vi "Binary-record-&-read.vi"   [LabVIEW 2015]
uses:
  <vilib>/Platform/TimedLoop/XDataNode/timing_clust.ctl
  <vilib>/Platform/TimedLoop/XDataNode/nitl_modes.ctl
  <vilib>/Platform/TimedLoop/XDataNode/wakeup.ctl
  <vilib>/Rock Robotics/WPI/Utilities/WPI_GetSetVariantRefNum.vi
  Robot Global Data.vi
  <vilib>/platform/TimedLoop/XDataNode/XDataNode.xnode
  <vilib>/Platform/TimedLoop/XDataNode/XDNodeRunTimeDep.lvlib
types:
  T1 = typedef "WPI_MotorControlDeviceRef.ctl" = cluster{"DeviceStatus":errorcluster, "Type":T2, "PWM":cluster{"PWM Channel":T3, "DeadBand":T4}, "CAN":cluster{"Device Number":u8, "Control Mode":T5, "Semaphore":T6, "Max Vout":dbl, "TalonSRX Control Mode":T7}, "Invert":bool}
  T2 = typedef "WPI_MotorControlType.ctl" = enum16{"PWM", "CAN", "CANTalonSRX"}
  T3 = typedef "FPGA_DIOPWMChannel.ctl" = enum8{"PWM 0", "PWM 1", "PWM 2", "PWM 3", "PWM 4", "PWM 5", "PWM 6", "PWM 7", "PWM 8", "PWM 9", "PWM MXP 0", "PWM MXP 1", "PWM MXP 2", "PWM MXP 3", "PWM MXP 4", "PWM MXP 5", "PWM MXP 6", "PWM MXP 7", "PWM MXP 8", "PWM MXP 9", "Invalid"}
  T4 = typedef "WPI_PWMDeadband.ctl" = cluster{"Name":string, "maxPositivePwm":i32, "minPositivePwm":i32, "centerPwm":i32, "maxNegativePwm":i32, "minNegativePwm":i32, "angularRange":u16}
  T5 = typedef "WPI_CANJaguar_ControlMode.ctl" = enum8{"Percent VBus", "Current", "Speed", "Position", "Voltage"}
  T6 = typedef "Semaphore RefNum" = refnum<k1>
  T7 = typedef "WPI_CANTalonSRX_APIControlMode.ctl" = enum8{"Percent VBus", "Speed", "Position", "Slave", "Unchanged / Invalid", "Voltage Compensation", "Current", "Motion Profile"}
  T8 = typedef "WPI_JoystickDevRef.ctl" = cluster{"Device":T9}
  T9 = typedef "WPI_JoystickDeviceEnum.ctl" = enum16{"USB 0", "USB 1", "USB 2", "USB 3", "USB 4", "USB 5"}
  T10 = typedef "XDNodeRunTimeDep.lvlib/timing_clust.ctl" = cluster{"Expected End [f-1]":u64, "Actual End [f-1]":u64, "Finished Late? [f-1]":bool, "Expected End [i-1]":u64, "Actual End [i-1]":u64, "Finished Late? [i-1]":bool, "Expected Start [i]":u64, "Actual Start [i]":u64, "Expected Start [f]":u64, "Actual Start [f]":u64, "Source Name":string, "Structure Name":string, "Period":i64, "Deadline":i64, "Offset":i64, "Start":i64, "Priority":i32, "Timeout":i32, "Mode":T11, "Wakeup Reason":T12, "Error":errorcluster, "Source Type":string, "Secondary Source Type":string, "Global End Time":u64, "Global Start Time":u64, "Frame Duration":u64, "Iteration Duration":u64, "Assigned CPU":i32, "I/O Scan Engine Mode":u32}
  T11 = typedef "XDNodeRunTimeDep.lvlib/nitl_modes.ctl" = enum32{"No Change", "Process missed periods, maintain original phase", "Discard missed periods, maintain original phase", "Process missed periods, ignore original phase", "Discard missed periods, ignore original phase"}
  T12 = typedef "XDNodeRunTimeDep.lvlib/wakeup.ctl" = enum32{"Normal", "Aborted", "Asynchronous wakeup", "Timing source error", "Timed loop error", "Timeout"}
  T13 = enum16{"open", "replace", "create", "open or create", "replace or create", "replace or create with confirmation"}
  T14 = enum16{"open", "open or create", "create or replace", "create", "open (read-only)"}
  T15 = cluster{"Record?":bool, "Current File":string, "Run script?":bool, "Stop recording?":bool, "Stop script?":bool}
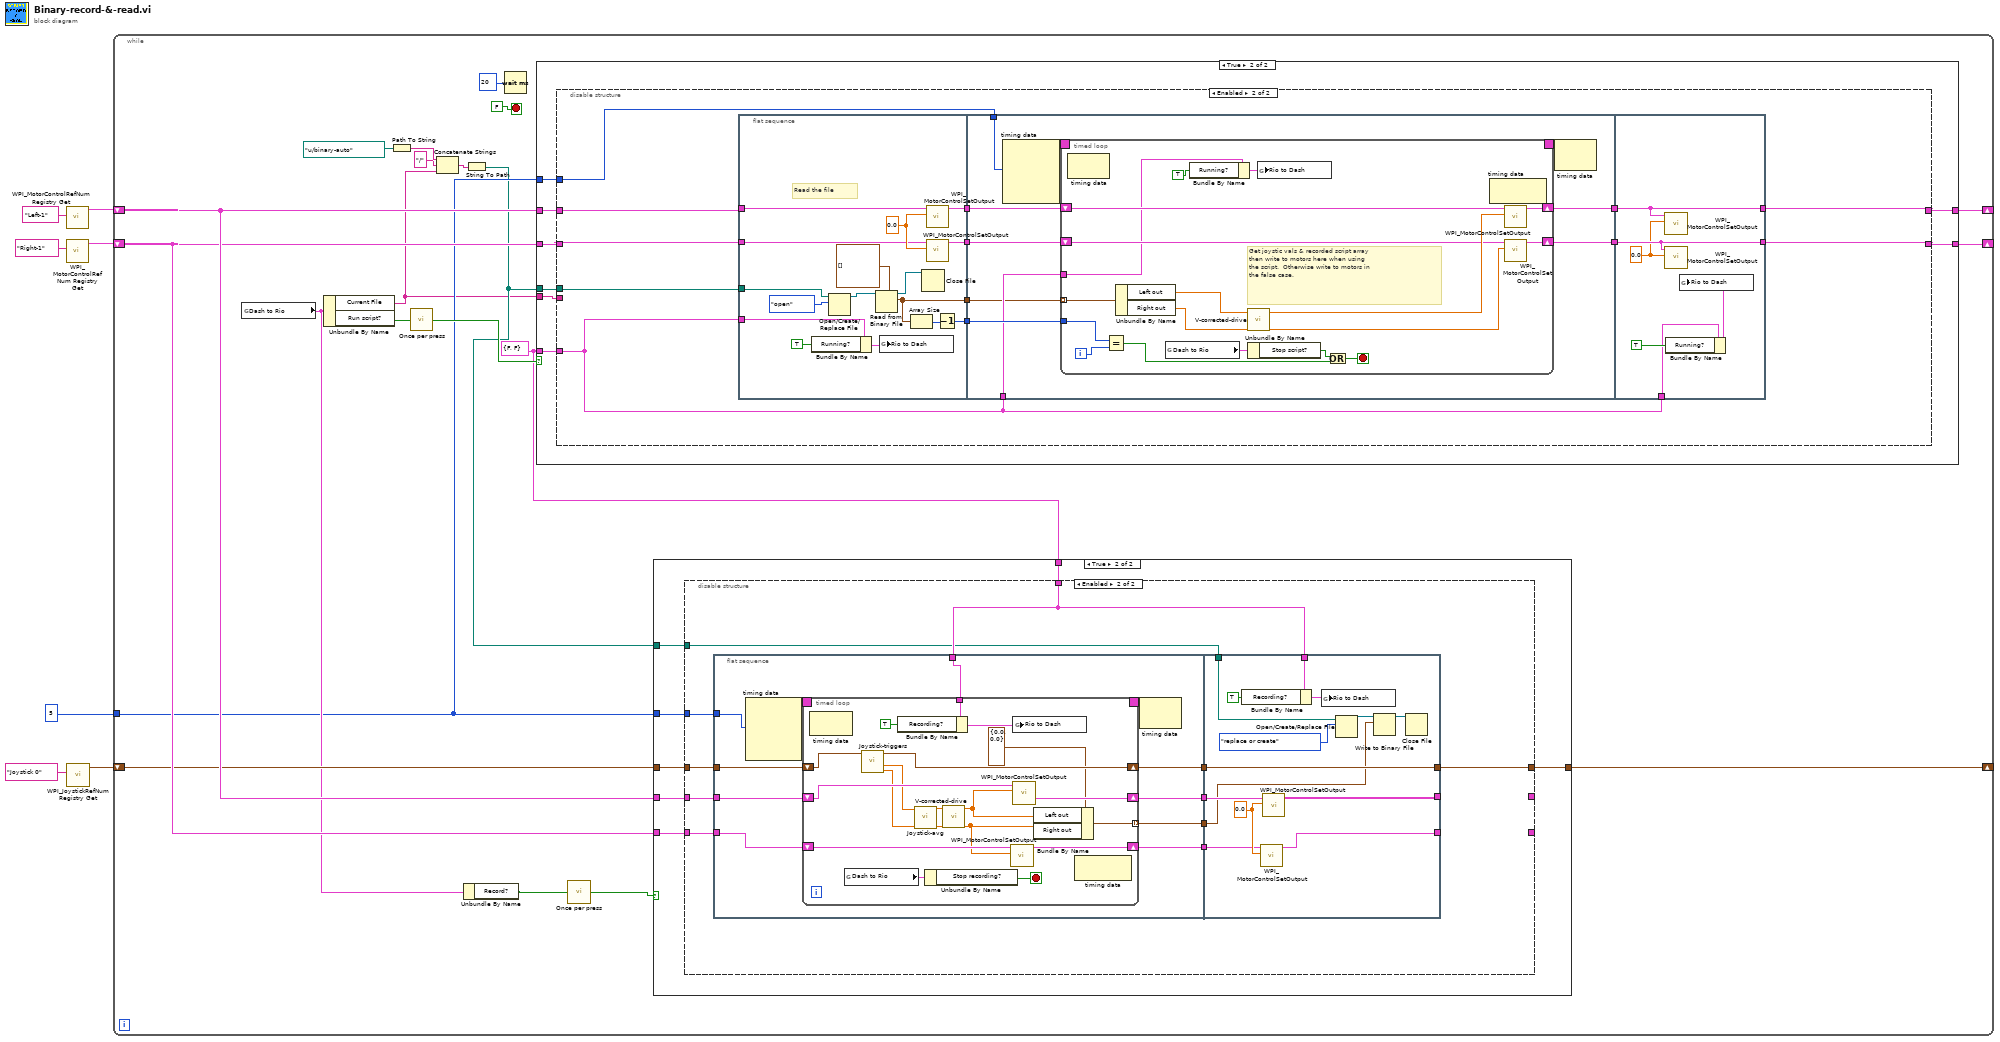
[diagram p0: block diagram]
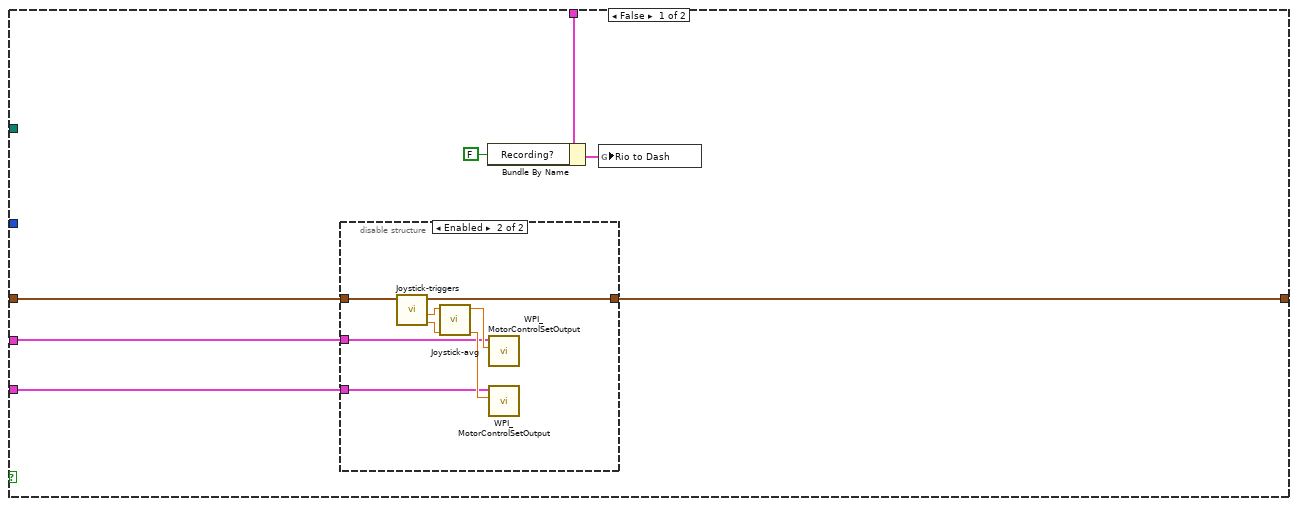
[diagram p2: hidden frame]
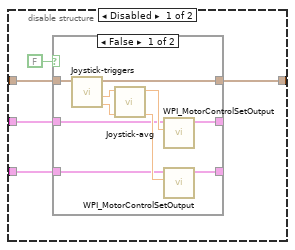
[diagram p3: hidden frame]
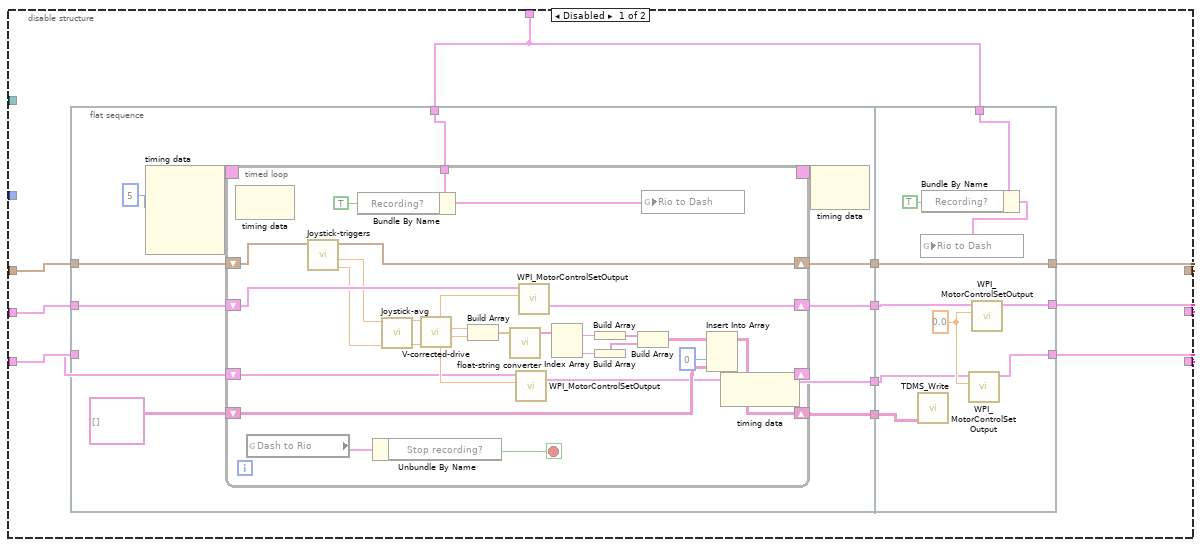
[diagram p5: hidden frame]
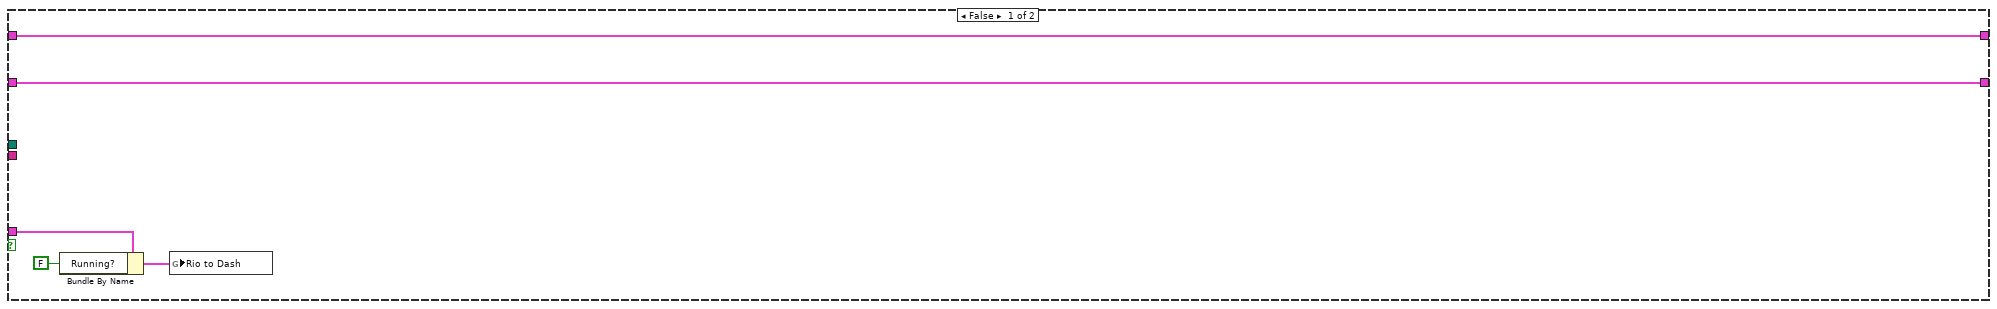
[diagram p6: hidden frame]
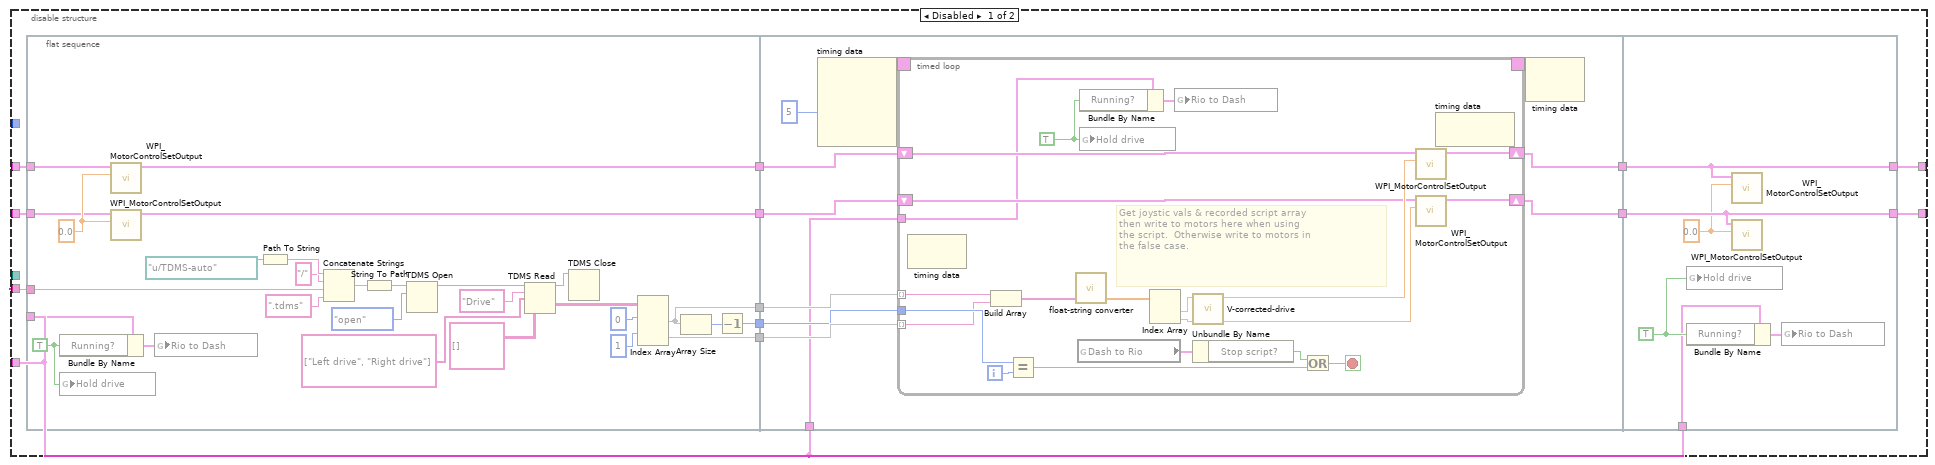
[diagram p7: hidden frame]
diagram:
  n1 = call <vilib>:"WPI_MotorControlRefNum Registry Get.vi"("refnum name"="Left-1") -> ("MotorControlDevRef"=w4:T1)  [unwired: 9 in, 1 out]
  n2 = call <vilib>:"WPI_MotorControlRefNum Registry Get.vi"("refnum name"="Right-1") -> ("MotorControlDevRef"=w5:T1)  [unwired: 9 in, 1 out]
  n3 = call <vilib>:"WPI_JoystickRefNum Registry Get.vi"("refnum name"="Joystick 0") -> ("JoystickDevRef"=w2:T8)  [unwired: 1 in, 9 out]
  n4 = while {
    shift-right: [w26] -> _
    shift-left: w5 -> [w20]
    shift-right: [w25] -> _
    shift-left: w4 -> [w21]
    shift-right: [w19] -> _
    shift-left: w2 -> [w18]
    tunnel: i64 5 ("Period") -> [w15]
    stop <- FALSE stop-if-true
    w16 = cluster{"Recording?":bool, "Running?":bool} {"Recording?"=FALSE, "Running?"=FALSE} ("Rio to Dash")
    n5 = global read "Robot Global Data.vi" "Dash to Rio"() -> (w17:T15)
    n6 = Unbundle By Name(w17) -> ("Current File"=w9:string, "Run script?"=w23:bool)
    n7 = Path To String(path=path "u:/binary-auto" ("file path 3")) -> (string=w13:string)
    n8 = call "Once per press.vi"("In"=w23) -> ("Out"=w24:bool)  [unwired: 2 in]
    n9 = Concatenate Strings(w13, "/" ("string"), w9) -> (w12:string)
    n10 = Unbundle By Name(w17) -> ("Record?"=w22:bool)
    n11 = String To Path(string=w12) -> (path=w10:path)
    n12 = Wait (ms)(milliseconds to wait=u32 20) -> ()  [unwired: 1 out]
    n13 = case shown="True" w24 {
      tunnel: w21 -> [w200 w208]
      tunnel: w20 -> [w199 w207]
      tunnel: [w200 w206] -> w25
      tunnel: [w199 w205] -> w26
      tunnel: w16 -> [w197 w204]
      tunnel: w15 -> [_ w203]
      tunnel: w10 -> [_ w202]
      tunnel: w9 -> [_ w201]
      frame False {
        n14 = Bundle By Name(cluster=w197, "Running?"=FALSE) -> (w198:cluster{"Recording?":bool, "Running?":bool})
        n15 = global write "Robot Global Data.vi" "Rio to Dash"(w198) -> ()
      }
      frame True {
        n16 = disable-structure shown="Enabled" {
          disable-tunnel: w208 -> [w214 w301]
          disable-tunnel: w207 -> [w213 w300]
          disable-tunnel: [w212 w297] -> w206
          disable-tunnel: [w211 w296] -> w205
          disable-tunnel: w201 -> [w210 _]
          disable-tunnel: w204 -> [w209 w298]
          disable-tunnel: w203 -> [_ w295]
          disable-tunnel: w202 -> [_ w294]
          frame Disabled {
            n17 = flat-sequence {
              tunnel: [w243] -> w221
              tunnel: [w241] -> w220
              tunnel: [w245] -> w219
              tunnel: [w239] -> w218
              tunnel: [w238] -> w217
              tunnel: w214 -> [w236]
              tunnel: w213 -> [w235]
              tunnel: w210 -> [w226]
              tunnel: w209 -> [w223]
              tunnel: w221 -> [w258]
              tunnel: w220 -> [w260]
              tunnel: w219 -> [w259]
              tunnel: w218 -> [w254]
              tunnel: w217 -> [w253]
              tunnel: [w252] -> w216
              tunnel: [w251] -> w215
              tunnel: w209 -> [w250]
              tunnel: w216 -> [w293]
              tunnel: w215 -> [w292]
              tunnel: [w293] -> w212
              tunnel: [w292] -> w211
              tunnel: w209 -> [w288]
              frame #0 {
                w222 = TRUE
                w237 = 0.0
                n18 = Bundle By Name(cluster=w223, "Running?"=w222) -> (w224:cluster{"Recording?":bool, "Running?":bool})
                n19 = global write "Robot Global Data.vi" "Hold drive"(w222) -> ()
                n20 = call <vilib>:"WPI_MotorControlSetOutput.vi"("Output"=w237, "MotorControlDevRef"=w236) -> ("MotorControlDevRef"=w239:T1)  [unwired: 7 in, 2 out]
                n21 = call <vilib>:"WPI_MotorControlSetOutput.vi"("Output"=w237, "MotorControlDevRef"=w235) -> ("MotorControlDevRef"=w238:T1)  [unwired: 7 in, 2 out]
                n22 = global write "Robot Global Data.vi" "Rio to Dash"(w224) -> ()
                n23 = Path To String(path=path "u:/TDMS-auto" ("file path 3")) -> (string=w231:string)
                n24 = Concatenate Strings(w231, "/" ("string"), w226, ".tdms" ("string")) -> (w230:string)
                n25 = String To Path(string=w230) -> (path=w233:path)
                n26 = TDMS Open(10:T14."open" ("operation (0:open)"), 11:w233) -> (3:w227:refnum<k34>)  [unwired: 5 in, 1 out]
                n27 = TDMS Read(0:w227, 5:"Drive" ("group name in"), 7:string[] ["Left drive", "Right drive"] ("channel name(s) in"), 12:string[][] [] ("array w/ subset deleted")) -> (4:w225:refnum<k34>, 10:w246:string[][])  [unwired: 4 in, 4 out]
                n28 = TDMS Close(11:w225) -> ()  [unwired: 1 in, 2 out]
                n29 = Index Array(array=w246, index (row) #1=0, index (row) #2=1 ("index (row)")) -> (element #1=w241:string[], element #2=w245:string[])  [unwired: 2 in]
                n30 = Array Size(array=w241) -> (size(s)=w240:i32)
                n31 = Decrement(x=w240) -> (x-1=w243:i32)
              }
              frame #1 {
                n32 = node-c288(i64 5 ("Period")) -> (w257:T10)  [unwired: 3 in]
                n33 = timed-loop {
                  tunnel: w260 -> [w276] mode=indexing
                  tunnel: w259 -> [w277] mode=indexing
                  tunnel: w258 -> [w280]
                  timing: w257 -> [_]
                  timing-out: [_] -> w256
                  shift-right: [w267] -> w252
                  shift-left: w254 -> [w269]
                  shift-right: [w266] -> w251
                  shift-left: w253 -> [w268]
                  tunnel: w250 -> [w261]
                  i -> [w281]
                  stop <- w279 stop-if-true
                  w262 = TRUE
                  # "Get joystic vals & recorded script array\nthen write to motors here when using\nthe script.  Otherwise write to motors in \nthe false case."
                  n34 = node-c288() -> ()  [unwired: 1 in, 1 out]
                  n35 = Build Array(w276, w277) -> (w275:string[])
                  n36 = Equal?(x=w280, y=w281) -> (x = y?=w278:bool)
                  n37 = call "float-string converter.vi"("float string in"=w275) -> ("float out"=w274:dbl[])  [unwired: 3 in, 1 out]
                  n38 = global read "Robot Global Data.vi" "Dash to Rio"() -> (w265:T15)
                  n39 = Bundle By Name(cluster=w261, "Running?"=w262) -> (w263:cluster{"Recording?":bool, "Running?":bool})
                  n40 = global write "Robot Global Data.vi" "Hold drive"(w262) -> ()
                  n41 = Index Array(array=w274) -> (element #1=w271:dbl, element #2=w270:dbl)  [unwired: 2 in]
                  n42 = global write "Robot Global Data.vi" "Rio to Dash"(w263) -> ()
                  n43 = call "V-corrected-drive.vi"("R-IN"=w270, "L-IN 2"=w271) -> ("Right out"=w273:dbl, "Left out"=w272:dbl)  [unwired: 8 in]
                  n44 = Unbundle By Name(w265) -> ("Stop script?"=w264:bool)
                  n45 = Or(x=w264, y=w278) -> (x .or. y?=w279:bool)
                  n46 = call <vilib>:"WPI_MotorControlSetOutput.vi"("Output"=w272, "MotorControlDevRef"=w269) -> ("MotorControlDevRef"=w267:T1)  [unwired: 7 in, 2 out]
                  n47 = call <vilib>:"WPI_MotorControlSetOutput.vi"("Output"=w273, "MotorControlDevRef"=w268) -> ("MotorControlDevRef"=w266:T1)  [unwired: 7 in, 2 out]
                  n48 = node-c288() -> ()  [unwired: 1 in, 1 out]
                }
                n49 = node-c288(w256) -> ()  [unwired: 1 out]
              }
              frame #2 {
                w289 = TRUE
                w291 = 0.0
                n50 = global write "Robot Global Data.vi" "Hold drive"(w289) -> ()
                n51 = Bundle By Name(cluster=w288, "Running?"=w289) -> (w290:cluster{"Recording?":bool, "Running?":bool})
                n52 = call <vilib>:"WPI_MotorControlSetOutput.vi"("Output"=w291, "MotorControlDevRef"=w293) -> ()  [unwired: 7 in, 3 out]
                n53 = call <vilib>:"WPI_MotorControlSetOutput.vi"("Output"=w291, "MotorControlDevRef"=w292) -> ()  [unwired: 7 in, 3 out]
                n54 = global write "Robot Global Data.vi" "Rio to Dash"(w290) -> ()
              }
            }
          }
          frame Enabled {
            n55 = flat-sequence {
              tunnel: [w322] -> w306
              tunnel: [w320] -> w305
              tunnel: [w319] -> w304
              tunnel: w301 -> [w317]
              tunnel: w300 -> [w316]
              tunnel: w298 -> [w314]
              tunnel: [w308] -> w299
              tunnel: w294 -> [w307]
              tunnel: w306 -> [w332]
              tunnel: w305 -> [w329]
              tunnel: w304 -> [w328]
              tunnel: [w327] -> w303
              tunnel: [w326] -> w302
              tunnel: w298 -> [w325]
              tunnel: w299 -> [w324]
              tunnel: w295 -> [w323]
              tunnel: w303 -> [w362]
              tunnel: w302 -> [w361]
              tunnel: [w362] -> w297
              tunnel: [w361] -> w296
              tunnel: w298 -> [w357]
              frame #0 {
                w318 = 0.0
                # "Read the file"
                n56 = Bundle By Name(cluster=w314, "Running?"=TRUE) -> (w315:cluster{"Recording?":bool, "Running?":bool})
                n57 = Open/Create/Replace File(file path (use dialog)=w307, operation (0:open)=T13."open") -> (refnum out=w311:refnum<file>)  [unwired: 4 in, 2 out]
                n58 = Read from Binary File(5:cluster{"Left out":dbl, "Right out":dbl}[] [], 11:w311) -> (2:w308:cluster{"Left out":dbl, "Right out":dbl}[], 3:w309:refnum<file>)  [unwired: 4 in, 2 out]
                n59 = global write "Robot Global Data.vi" "Rio to Dash"(w315) -> ()
                n60 = Array Size(array=w308) -> (size(s)=w321:i32)
                n61 = Close File(refnum=w309) -> ()  [unwired: 1 in, 2 out]
                n62 = call <vilib>:"WPI_MotorControlSetOutput.vi"("Output"=w318, "MotorControlDevRef"=w317) -> ("MotorControlDevRef"=w320:T1)  [unwired: 7 in, 2 out]
                n63 = call <vilib>:"WPI_MotorControlSetOutput.vi"("Output"=w318, "MotorControlDevRef"=w316) -> ("MotorControlDevRef"=w319:T1)  [unwired: 7 in, 2 out]
                n64 = Decrement(x=w321) -> (x-1=w322:i32)
              }
              frame #1 {
                n65 = node-c288(w323) -> (w331:T10)  [unwired: 3 in]
                n66 = timed-loop {
                  tunnel: w332 -> [w349]
                  timing: w331 -> [_]
                  timing-out: [_] -> w330
                  shift-right: [w342] -> w327
                  shift-left: w329 -> [w344]
                  shift-right: [w341] -> w326
                  shift-left: w328 -> [w343]
                  tunnel: w325 -> [w333]
                  tunnel: w324 -> [w336] mode=indexing
                  i -> [w350]
                  stop <- w348 stop-if-true
                  # "Get joystic vals & recorded script array\nthen write to motors here when using\nthe script.  Otherwise write to motors in \nthe false case."
                  n67 = node-c288() -> ()  [unwired: 1 in, 1 out]
                  n68 = Equal?(x=w349, y=w350) -> (x = y?=w347:bool)
                  n69 = Unbundle By Name(w336) -> ("Left out"=w335:dbl, "Right out"=w334:dbl)
                  n70 = global read "Robot Global Data.vi" "Dash to Rio"() -> (w340:T15)
                  n71 = Bundle By Name(cluster=w333, "Running?"=TRUE) -> (w338:cluster{"Recording?":bool, "Running?":bool})
                  n72 = call "V-corrected-drive.vi"("R-IN"=w334, "L-IN 2"=w335) -> ("Right out"=w346:dbl, "Left out"=w345:dbl)  [unwired: 8 in]
                  n73 = Unbundle By Name(w340) -> ("Stop script?"=w339:bool)
                  n74 = global write "Robot Global Data.vi" "Rio to Dash"(w338) -> ()
                  n75 = Or(x=w339, y=w347) -> (x .or. y?=w348:bool)
                  n76 = node-c288() -> ()  [unwired: 1 in, 1 out]
                  n77 = call <vilib>:"WPI_MotorControlSetOutput.vi"("Output"=w345, "MotorControlDevRef"=w344) -> ("MotorControlDevRef"=w342:T1)  [unwired: 7 in, 2 out]
                  n78 = call <vilib>:"WPI_MotorControlSetOutput.vi"("Output"=w346, "MotorControlDevRef"=w343) -> ("MotorControlDevRef"=w341:T1)  [unwired: 7 in, 2 out]
                }
                n79 = node-c288(w330) -> ()  [unwired: 1 out]
              }
              frame #2 {
                w360 = 0.0
                n80 = call <vilib>:"WPI_MotorControlSetOutput.vi"("Output"=w360, "MotorControlDevRef"=w362) -> ()  [unwired: 7 in, 3 out]
                n81 = call <vilib>:"WPI_MotorControlSetOutput.vi"("Output"=w360, "MotorControlDevRef"=w361) -> ()  [unwired: 7 in, 3 out]
                n82 = Bundle By Name(cluster=w357, "Running?"=TRUE) -> (w359:cluster{"Recording?":bool, "Running?":bool})
                n83 = global write "Robot Global Data.vi" "Rio to Dash"(w359) -> ()
              }
            }
          }
        }
      }
    }
    n84 = call "Once per press.vi"("In"=w22) -> ("Out"=w8:bool)  [unwired: 2 in]
    n85 = case shown="True" w8 {
      tunnel: w18 -> [w35 w68]
      tunnel: w21 -> [w34 w67]
      tunnel: w20 -> [w33 w66]
      tunnel: w16 -> [w31 w65]
      tunnel: [w29 w64] -> w19
      tunnel: w15 -> [_ w63]
      tunnel: w10 -> [_ w62]
      frame False {
        n86 = disable-structure shown="Enabled" {
          disable-tunnel: w35 -> [w40 w57]
          disable-tunnel: w34 -> [w39 w56]
          disable-tunnel: w33 -> [w38 w55]
          disable-tunnel: [w37 w54] -> w29
          frame Disabled {
            n87 = case shown="False" FALSE {
              tunnel: w40 -> [w48 w53]
              tunnel: [w47 w53] -> w37
              tunnel: [w44 w51] -> _
              tunnel: [w43 w52] -> _
              tunnel: w39 -> [w42 w52]
              tunnel: w38 -> [w41 w51]
              frame False {
                n88 = call "Joystick-triggers.vi"("JoystickDevRef"=w48) -> ("Right out"=w49:dbl, "Left out"=w50:dbl, "JoystickDevRef out"=w47:T8)  [unwired: 6 in, 2 out]
                n89 = call "Joystick-avg.vi"("Joystic right axis in"=w49, "Joystic left axis in"=w50) -> ("Right out"=w45:dbl, "Left out"=w46:dbl)  [unwired: 8 in]
                n90 = call <vilib>:"WPI_MotorControlSetOutput.vi"("Output"=w46, "MotorControlDevRef"=w42) -> ("MotorControlDevRef"=w43:T1)  [unwired: 7 in, 2 out]
                n91 = call <vilib>:"WPI_MotorControlSetOutput.vi"("Output"=w45, "MotorControlDevRef"=w41) -> ("MotorControlDevRef"=w44:T1)  [unwired: 7 in, 2 out]
              }
              frame True {
              }
            }
          }
          frame Enabled {
            n92 = call "Joystick-triggers.vi"("JoystickDevRef"=w57) -> ("Right out"=w60:dbl, "Left out"=w61:dbl, "JoystickDevRef out"=w54:T8)  [unwired: 6 in, 2 out]
            n93 = call "Joystick-avg.vi"("Joystic right axis in"=w60, "Joystic left axis in"=w61) -> ("Right out"=w58:dbl, "Left out"=w59:dbl)  [unwired: 8 in]
            n94 = call <vilib>:"WPI_MotorControlSetOutput.vi"("Output"=w59, "MotorControlDevRef"=w56) -> ()  [unwired: 7 in, 3 out]
            n95 = call <vilib>:"WPI_MotorControlSetOutput.vi"("Output"=w58, "MotorControlDevRef"=w55) -> ()  [unwired: 7 in, 3 out]
          }
        }
        n96 = Bundle By Name(cluster=w31, "Recording?"=FALSE) -> (w32:cluster{"Recording?":bool, "Running?":bool})
        n97 = global write "Robot Global Data.vi" "Rio to Dash"(w32) -> ()
      }
      frame True {
        n98 = disable-structure shown="Enabled" {
          disable-tunnel: w68 -> [w75 w142]
          disable-tunnel: w67 -> [w74 w141]
          disable-tunnel: w66 -> [w73 w140]
          disable-tunnel: [w72 w137] -> w64
          disable-tunnel: [w71 _] -> _
          disable-tunnel: [w70 _] -> _
          disable-tunnel: w65 -> [w69 w139]
          disable-tunnel: w63 -> [_ w136]
          disable-tunnel: w62 -> [_ w135]
          frame Disabled {
            n99 = flat-sequence {
              tunnel: [w87] -> w79
              tunnel: w75 -> [w86]
              tunnel: w74 -> [w85]
              tunnel: w73 -> [w84]
              tunnel: [w83] -> w78
              tunnel: [w82] -> w77
              tunnel: [w81] -> w76
              tunnel: w69 -> [w80]
              tunnel: w79 -> [w134]
              tunnel: w78 -> [w132]
              tunnel: w77 -> [w131]
              tunnel: [w130] -> w72
              tunnel: w76 -> [w130]
              tunnel: [w129] -> w71
              tunnel: [w128] -> w70
              tunnel: w69 -> [w127]
              frame #0 {
                n100 = node-c288(i64 5 ("Period")) -> (w91:T10)  [unwired: 3 in]
                n101 = timed-loop {
                  timing: w91 -> [_]
                  timing-out: [_] -> w90
                  shift-right: [w109] -> w87
                  shift-left: string[][] [] -> [w110]
                  shift-right: [w103] -> w82
                  shift-left: w84 -> [w104]
                  shift-right: [w101] -> w83
                  shift-left: w85 -> [w102]
                  shift-right: [w99] -> w81
                  shift-left: w86 -> [w100]
                  tunnel: w80 -> [w92]
                  stop <- w95 stop-if-true
                  n102 = node-c288() -> ()  [unwired: 1 in, 1 out]
                  n103 = global read "Robot Global Data.vi" "Dash to Rio"() -> (w96:T15)
                  n104 = call "Joystick-triggers.vi"("JoystickDevRef"=w100) -> ("Right out"=w97:dbl, "Left out"=w98:dbl, "JoystickDevRef out"=w99:T8)  [unwired: 6 in, 2 out]
                  n105 = Bundle By Name(cluster=w92, "Recording?"=TRUE) -> (w93:cluster{"Recording?":bool, "Running?":bool})
                  n106 = Unbundle By Name(w96) -> ("Stop recording?"=w95:bool)
                  n107 = call "Joystick-avg.vi"("Joystic right axis in"=w97, "Joystic left axis in"=w98) -> ("Right out"=w107:dbl, "Left out"=w108:dbl)  [unwired: 8 in]
                  n108 = call "V-corrected-drive.vi"("R-IN"=w107, "L-IN 2"=w108) -> ("Right out"=w106:dbl, "Left out"=w105:dbl)  [unwired: 8 in]
                  n109 = Build Array(w105, w106) -> (w114:dbl[])
                  n110 = call "float-string converter.vi"("float in"=w114) -> ("float string out"=w113:string[])  [unwired: 3 in, 1 out]
                  n111 = call <vilib>:"WPI_MotorControlSetOutput.vi"("Output"=w106, "MotorControlDevRef"=w104) -> ("MotorControlDevRef"=w103:T1)  [unwired: 7 in, 2 out]
                  n112 = call <vilib>:"WPI_MotorControlSetOutput.vi"("Output"=w105, "MotorControlDevRef"=w102) -> ("MotorControlDevRef"=w101:T1)  [unwired: 7 in, 2 out]
                  n113 = Index Array(array=w113) -> (element #1=w112:string, element #2=w111:string)  [unwired: 2 in]
                  n114 = Build Array(w112) -> (w117:string[])
                  n115 = Build Array(w111) -> (w118:string[])
                  n116 = Build Array(w117, w118) -> (w116:string[][])
                  n117 = global write "Robot Global Data.vi" "Rio to Dash"(w93) -> ()
                  n118 = Insert Into Array(array=w116, index (col)=0 ("disabled index (col)"), new element=w110) -> (w109:string[][])  [unwired: 1 in]
                  n119 = node-c288() -> ()  [unwired: 1 in, 1 out]
                }
                n120 = node-c288(w90) -> ()  [unwired: 1 out]
              }
              frame #1 {
                w133 = 0.0 ("Output")
                n121 = call "TDMS_Write.vi"("2D data array"=w134) -> ()  [unwired: 11 in]
                n122 = Bundle By Name(cluster=w127, "Recording?"=TRUE) -> (w125:cluster{"Recording?":bool, "Running?":bool})
                n123 = global write "Robot Global Data.vi" "Rio to Dash"(w125) -> ()
                n124 = call <vilib>:"WPI_MotorControlSetOutput.vi"("Output"=w133, "MotorControlDevRef"=w131) -> ("MotorControlDevRef"=w128:T1)  [unwired: 7 in, 2 out]
                n125 = call <vilib>:"WPI_MotorControlSetOutput.vi"("Output"=w133, "MotorControlDevRef"=w132) -> ("MotorControlDevRef"=w129:T1)  [unwired: 7 in, 2 out]
              }
            }
          }
          frame Enabled {
            n126 = flat-sequence {
              tunnel: w142 -> [w154]
              tunnel: w141 -> [w153]
              tunnel: w140 -> [w152]
              tunnel: [w151] -> w145
              tunnel: [w150] -> w144
              tunnel: [w149] -> w143
              tunnel: w139 -> [w148]
              tunnel: [w147] -> w138
              tunnel: w136 -> [w146]
              tunnel: w145 -> [w194]
              tunnel: w144 -> [w193]
              tunnel: [w192] -> w137
              tunnel: w143 -> [w192]
              tunnel: [w191] -> _
              tunnel: [w190] -> _
              tunnel: w139 -> [w189]
              tunnel: w138 -> [w183]
              tunnel: w135 -> [w182]
              frame #0 {
                n127 = node-c288(w146) -> (w156:T10)  [unwired: 3 in]
                n128 = timed-loop {
                  timing: w156 -> [_]
                  timing-out: [_] -> w155
                  shift-right: [w172] -> w150
                  shift-left: w152 -> [w173]
                  shift-right: [w170] -> w151
                  shift-left: w153 -> [w171]
                  shift-right: [w168] -> w149
                  shift-left: w154 -> [w169]
                  tunnel: w148 -> [w161]
                  tunnel: [w158] -> w147 mode=indexing
                  stop <- w164 stop-if-true
                  n129 = node-c288() -> ()  [unwired: 1 in, 1 out]
                  n130 = global read "Robot Global Data.vi" "Dash to Rio"() -> (w165:T15)
                  n131 = call "Joystick-triggers.vi"("JoystickDevRef"=w169) -> ("Right out"=w166:dbl, "Left out"=w167:dbl, "JoystickDevRef out"=w168:T8)  [unwired: 6 in, 2 out]
                  n132 = Bundle By Name(cluster=w161, "Recording?"=TRUE) -> (w162:cluster{"Recording?":bool, "Running?":bool})
                  n133 = call "Joystick-avg.vi"("Joystic right axis in"=w166, "Joystic left axis in"=w167) -> ("Right out"=w174:dbl, "Left out"=w175:dbl)  [unwired: 8 in]
                  n134 = Unbundle By Name(w165) -> ("Stop recording?"=w164:bool)
                  n135 = call "V-corrected-drive.vi"("R-IN"=w174, "L-IN 2"=w175) -> ("Right out"=w159:dbl, "Left out"=w160:dbl)  [unwired: 8 in]
                  n136 = call <vilib>:"WPI_MotorControlSetOutput.vi"("Output"=w159, "MotorControlDevRef"=w173) -> ("MotorControlDevRef"=w172:T1)  [unwired: 7 in, 2 out]
                  n137 = global write "Robot Global Data.vi" "Rio to Dash"(w162) -> ()
                  n138 = call <vilib>:"WPI_MotorControlSetOutput.vi"("Output"=w160, "MotorControlDevRef"=w171) -> ("MotorControlDevRef"=w170:T1)  [unwired: 7 in, 2 out]
                  n139 = Bundle By Name(cluster=cluster{"Left out":dbl, "Right out":dbl} {"Left out"=0.0, "Right out"=0.0}, "Left out"=w160, "Right out"=w159) -> (w158:cluster{"Left out":dbl, "Right out":dbl})
                  n140 = node-c288() -> ()  [unwired: 1 in, 1 out]
                }
                n141 = node-c288(w155) -> ()  [unwired: 1 out]
              }
              frame #1 {
                w195 = 0.0 ("Output")
                n142 = Bundle By Name(cluster=w189, "Recording?"=TRUE) -> (w187:cluster{"Recording?":bool, "Running?":bool})
                n143 = call <vilib>:"WPI_MotorControlSetOutput.vi"("Output"=w195, "MotorControlDevRef"=w193) -> ("MotorControlDevRef"=w190:T1)  [unwired: 7 in, 2 out]
                n144 = call <vilib>:"WPI_MotorControlSetOutput.vi"("Output"=w195, "MotorControlDevRef"=w194) -> ("MotorControlDevRef"=w191:T1)  [unwired: 7 in, 2 out]
                n145 = global write "Robot Global Data.vi" "Rio to Dash"(w187) -> ()
                n146 = Open/Create/Replace File(file path (use dialog)=w182, operation (0:open)=T13."replace or create") -> (refnum out=w185:refnum<file>)  [unwired: 4 in, 2 out]
                n147 = Write to Binary File(file (use dialog)=w185, data=w183) -> (refnum out=w186:refnum<file>)  [unwired: 4 in, 2 out]
                n148 = Close File(refnum=w186) -> ()  [unwired: 1 in, 2 out]
              }
            }
          }
        }
      }
    }
  }
